vi "RP Read Subset.vi"   [LabVIEW 2019]
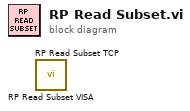
[diagram p0: block diagram]
diagram:
  n1 = call "RP Read Subset VISA.vi"() -> ()  [unwired: 8 in, 4 out]
  n2 = call "RP Read Subset TCP.vi"() -> ()  [unwired: 8 in, 4 out]
